vi "setICCamAcq.vi"(8 "error in (no error)":errorcluster, 10 "ICCameraAcquisitor":refnum<class "ICCameraAcquisitor.lvclass">, 11 "ICCameraController in":refnum<class "ICCameraController.lvclass">) -> (0 "error out":errorcluster, 3 "ICCameraController out":refnum<class "ICCameraController.lvclass">)   [LabVIEW 2011, in "Hardware.lvlib" / "Channels.lvlib" / "ICCameraController.lvclass"]
uses:
  ICCameraController.lvclass
  ICCameraAcquisitor/ICCameraAcquisitor.lvclass
  ICCameraController.lvclass/ICCameraController.ctl
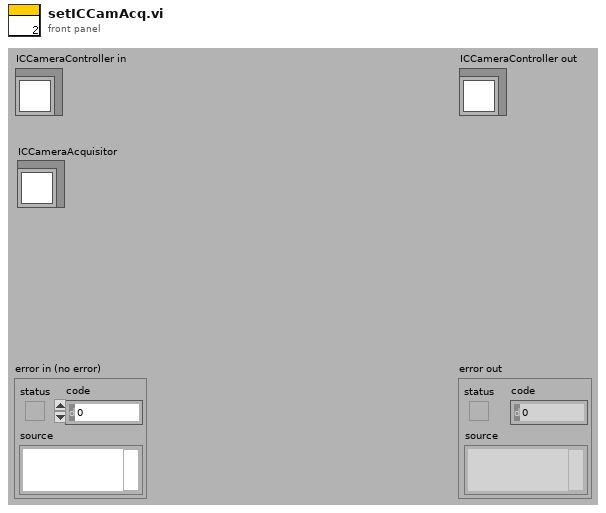
[diagram p1: front panel]
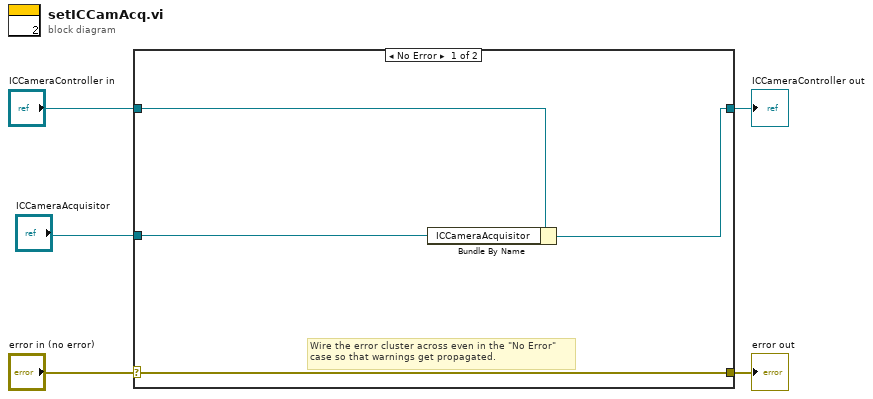
[diagram p0: block diagram]
diagram:
  n1 = case shown="No Error" "error in (no error)" {
    selector: "error in (no error)" -> [w9 w11]
    tunnel: [w9 w11] -> w4
    tunnel: [w7 w10] -> w2
    tunnel: "ICCameraController in" -> [w8 w10]
    tunnel: "ICCameraAcquisitor" -> [w6 _]
    frame No Error {
      # "Wire the error cluster across even in the \"No Error\"\ncase so that warnings get propagated."
      n2 = Bundle By Name(cluster=w8, "ICCameraAcquisitor"=w6) -> (w7:refnum<class "ICCameraController.lvclass">)
    }
    frame Error {
    }
  }
  "error out" <- w4
  "ICCameraController out" <- w2
